vi "SQL Build Delete Query.vi"(8 "error in (no error)":errorcluster, 10 "condition":string, 11 "table":string) -> (0 "error out":errorcluster, 3 "Delect":string)   [LabVIEW 2011]
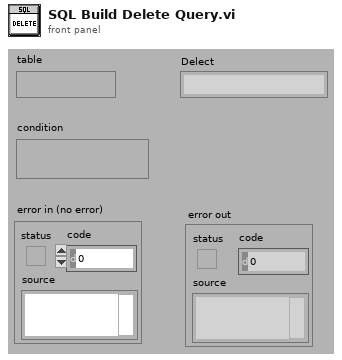
[diagram p1: front panel]
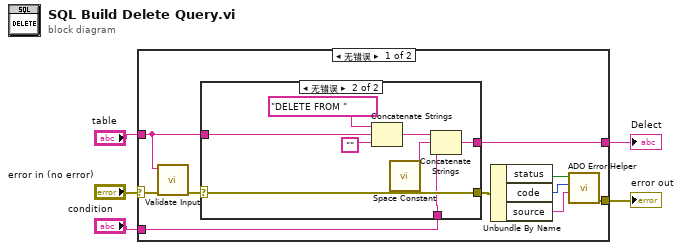
[diagram p0: block diagram]
diagram:
  n1 = case shown="无错误" "error in (no error)" {
    selector: "error in (no error)" -> [w8 w25]
    tunnel: [w11 w25] -> w2
    tunnel: "condition" -> [w10 _]
    tunnel: "table" -> [w9 _]
    tunnel: [w6 _] -> w1
    frame No Error {
      n2 = call "Validate Input.vi"("error in (no error)"=w8, "table"=w9) -> ("error out"=w7:errorcluster)  [unwired: 7 in, 2 out]
      n3 = case shown="无错误" w7 {
        selector: w7 -> [w16 w18]
        tunnel: [w16 w18] -> w12
        tunnel: w10 -> [_ w17]
        tunnel: w9 -> [_ w21]
        tunnel: [_ w19] -> w6
        frame Error {
          # "No table is specified; output error."
        }
        frame No Error {
          n4 = Concatenate Strings("DELETE FROM " ("Substring"), w21, "") -> (w20:string)
          n5 = call <vilib>:"Space Constant.vi"() -> ("String"=w24:string)
          n6 = Concatenate Strings(w20, w24, w17) -> (w19:string)
        }
      }
      n7 = Unbundle By Name(w12) -> ("status"=w15:bool, "code"=w14:i32, "source"=w13:string)
      n8 = call "ADO Error Helper.vi"("source"=w13, "code"=w14, "status"=w15) -> ("error out"=w11:errorcluster)  [unwired: 8 in]
    }
    frame Error {
    }
  }
  "error out" <- w2
  "Delect" <- w1
